vi "Locate Corner.vi"(7 "picture":refnum<vi>, 8 "error in":errorcluster, 9 "Corner Type":T1, 10 "Height":dbl=10000.0, 11 "color":string="Mat") -> (0 "error out":errorcluster, 2 "Robot Pose":cluster{"X":dbl, "Y":dbl, "Z":dbl, "A":dbl}, 3 "Robot Point":dbl[](array[numeric]), 5 "picture":picture)   [LabVIEW 2013]
uses:
  Teach Locations.ctl
  ROS/Code/SubVIs/BaxterSide.ctl
  <vilib>/Analysis/Matrix/Datatypes/RealMatrix.ctl
  <vilib>/Analysis/baseanly.llb/Mean (DBL).vi
  Arm Globals.vi
  Prim/Fwd Kenimatics - array.vi
  <vilib>/Analysis/Matrix/Numeric/Multiply/Multiply - RM,RM.vi
  ROS/Code/Console/Servers/ServerSubs/(nist) Arm Globals.vi
  Move/Move Axis.vi
  <vilib>/Analysis/Matrix/NI_Matrix.lvlib
  <vilib>/Analysis/NI_AALBase.lvlib
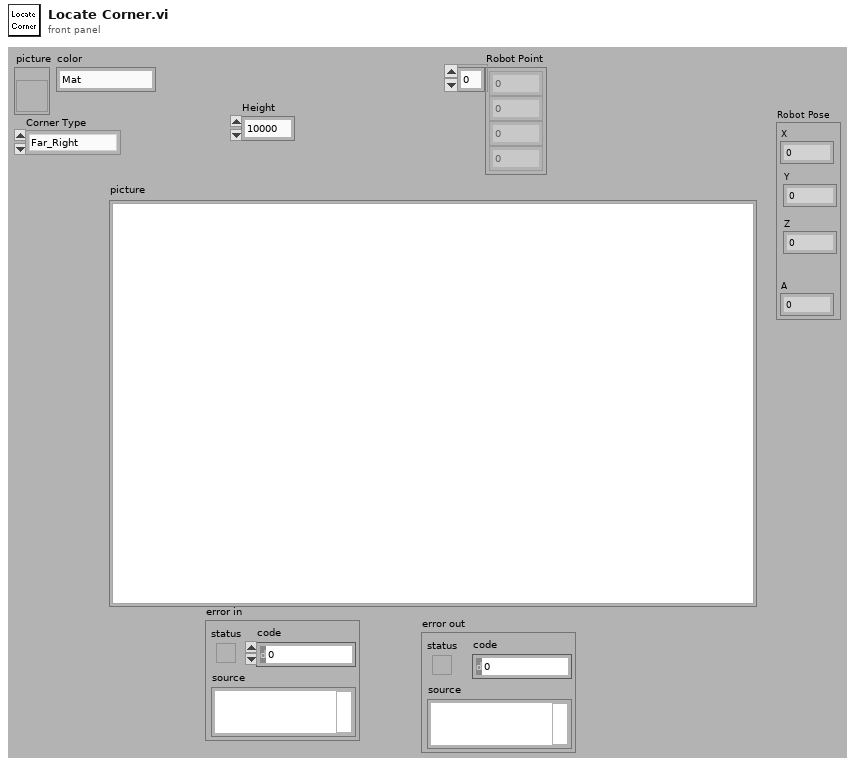
[diagram p1: front panel]
types:
  T1 = typedef "Teach Locations.ctl" = enum16{"Far_Right", "Near_Right", "Far_Left", "Near_Left", "Bottom", "Top", "Right", "Left"}
  T2 = cluster{"X":dbl, "Y":dbl, "Z":dbl, "O":dbl, "A":dbl, "T":dbl}
  T3 = typedef "BaxterSide.ctl" = enum16{"left", "right"}
  T4 = typedef "NI_Matrix.lvlib/RealMatrix.ctl" = dbl[][]
  T5 = cluster{"Real Matrix Element":dbl, "Real Matrix Element":dbl, "Real Matrix Element":dbl, "Real Matrix Element":dbl}
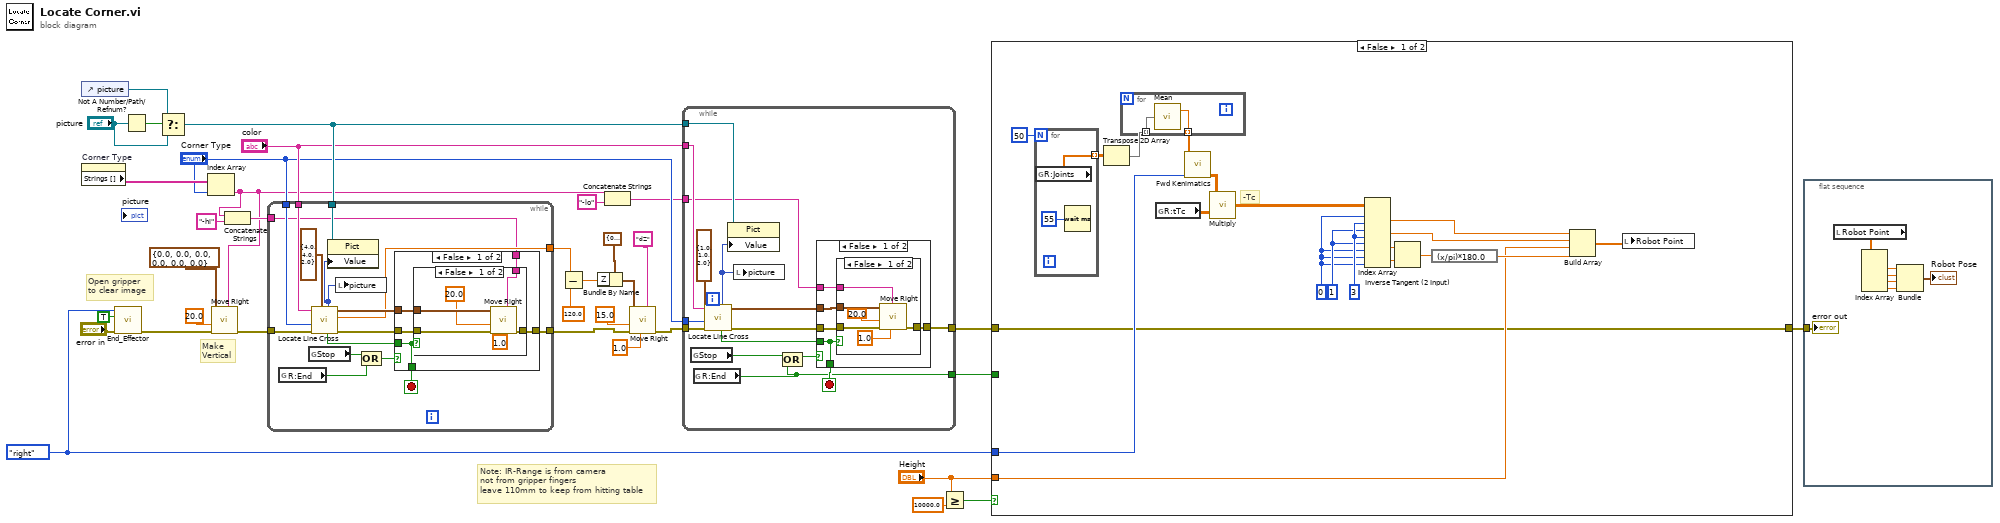
[diagram p0: block diagram]
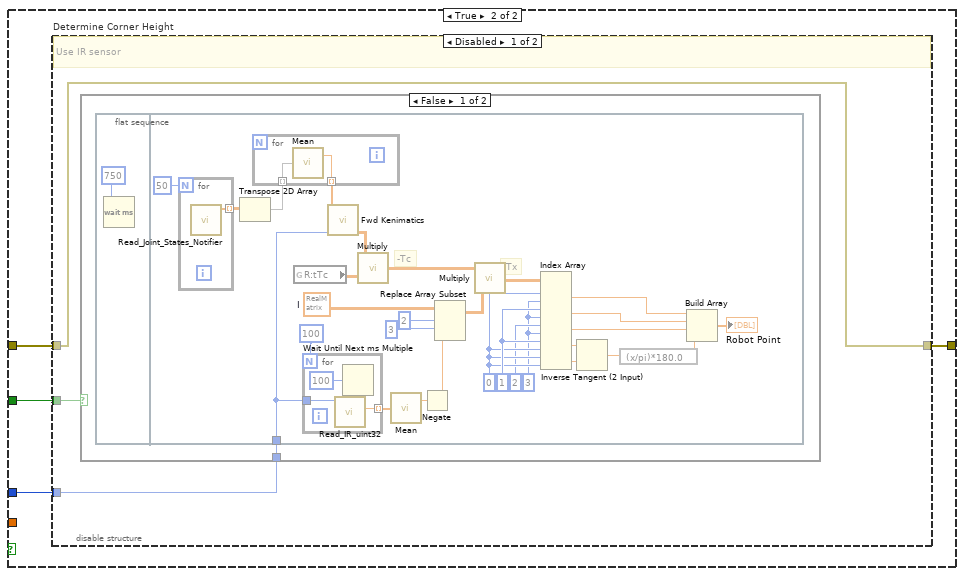
[diagram p2: hidden frame]
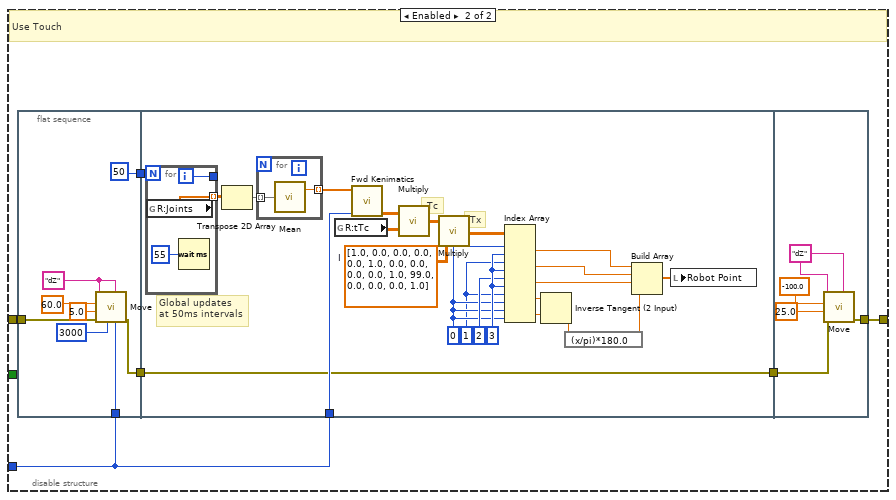
[diagram p4: hidden frame]
diagram:
  w23 = BaxterSide."right" ("Side")
  # "Make\nVertical"
  # "Open gripper\nto clear image"
  # "Note: IR-Range is from camera \nnot from gripper fingers\nleave 110mm to keep from hitting table"
  n1 = control-ref of="picture"() -> (w32:refnum<vi>)
  n2 = property on="Corner Type" class="Enum (strict)"() -> ("Strings []"=w25:string[])  [unwired: 2 in, 2 out]
  n3 = call "End_Effector.vi"("error in"="error in", "Close"=TRUE, "Side"=w23) -> ("error out"=w13:errorcluster)  [unwired: 5 in]
  n4 = Not A Number/Path/Refnum?(number/path/refnum="picture") -> (NaN/Path/Refnum?=w34:bool)
  n5 = Select(t=w32, s=w34, f="picture") -> (s? t:f=w35:refnum<vi>)
  n6 = Index Array(array=w25, index="Corner Type") -> (element=w10:string)
  n7 = call "Move Right.vi"("Label"=w10, "error in"=w13, "Speed (mm/s)"=20.0 ("Speed"), "Goal Axes"=T2 {"X"=0.0, "Y"=0.0, "Z"=0.0, "O"=0.0, "A"=0.0, "T"=0.0}) -> ("error out"=w12:errorcluster)  [unwired: 7 in]
  n8 = Concatenate Strings(w10, "-hi" ("string")) -> (w21:string)
  n9 = while {
    tunnel: w12 -> [w51]
    tunnel: [w49] -> w7
    tunnel: "color" -> [w39]
    tunnel: w35 -> [w43]
    tunnel: [w41] -> w27
    tunnel: "Corner Type" -> [w40]
    tunnel: w21 -> [w37]
    stop <- w45 stop-if-true
    n10 = global read "Arm Globals.vi" "R:End"() -> (w36:bool)
    n11 = global read "Arm Globals.vi" "Stop"() -> (w47:bool)
    n12 = call "Locate Line Cross.vi"("Tolerance"=cluster{"x":dbl, "y":dbl, "a":dbl} {"x"=4.0, "y"=4.0, "a"=2.0}, "error in"=w51, "Type"=w40, "color"=w39) -> ("error out"=w50:errorcluster, "Range"=w41:dbl, "result"=w48:T2, "Close"=w44:bool, "picture"=w38:picture)  [unwired: 2 in, 1 out]
    n13 = property class="Pict"(reference=w43, "Value"=w38) -> ()  [unwired: 1 in, 2 out]
    n14 = local write "picture"(w38) -> ()
    n15 = Compound Arithmetic op=OR(w47, w36) -> (w46:bool)
    n16 = case shown="False" w46 {
      selector: w46 -> [_ w64]
      tunnel: w50 -> [w56 w65]
      tunnel: [w55 w65] -> w49
      tunnel: w48 -> [w54 _]
      tunnel: [w53 w64] -> w45
      tunnel: w44 -> [w53 _]
      tunnel: w37 -> [w52 _]
      frame False {
        n17 = case shown="False" w53 {
          tunnel: w56 -> [w61 w63]
          tunnel: [w62 w63] -> w55
          tunnel: w54 -> [w58 _]
          tunnel: w52 -> [w60 _]
          frame False {
            n18 = call "Move Right.vi"("Label"=w60, "Wait Time"=1.0 ("wait time"), "error in"=w61, "Speed (mm/s)"=20.0 ("Speed"), "Goal Axes"=w58) -> ("error out"=w62:errorcluster)  [unwired: 6 in]
          }
          frame True {
          }
        }
      }
      frame True {
      }
    }
  }
  n19 = Subtract(x=w27, y=120.0) -> (x-y=w3:dbl)
  n20 = Bundle By Name(cluster=T2 {"X"=0.0, "Y"=0.0, "Z"=0.0, "O"=0.0, "A"=0.0, "T"=0.0} ("Goal Axes"), "Z"=w3) -> (w1:T2)
  n21 = Concatenate Strings(w10, "-lo" ("string")) -> (w19:string)
  n22 = call "Move Right.vi"("Label"="dZ" ("Location"), "Wait Time"=1.0 ("wait time"), "error in"=w7, "Speed (mm/s)"=15.0 ("Speed"), "Goal Axes"=w1) -> ("error out"=w8:errorcluster)  [unwired: 6 in]
  n23 = while {
    tunnel: w8 -> [w80]
    tunnel: [w78] -> w17
    tunnel: "color" -> [w75]
    tunnel: w35 -> [w71]
    tunnel: [w66] -> w29
    tunnel: "Corner Type" -> [w69]
    tunnel: w19 -> [w67]
    stop <- w72 stop-if-true
    n24 = global read "Arm Globals.vi" "Stop"() -> (w76:bool)
    n25 = global read "Arm Globals.vi" "R:End"() -> (w66:bool)
    n26 = call "Locate Line Cross.vi"("Tolerance"=cluster{"x":dbl, "y":dbl, "a":dbl} {"x"=1.0, "y"=1.0, "a"=2.0}, "error in"=w80, "Type"=w69, "color"=w75) -> ("error out"=w79:errorcluster, "result"=w77:T2, "Close"=w73:bool, "picture"=w68:picture)  [unwired: 2 in, 2 out]
    n27 = property class="Pict"(reference=w71, "Value"=w68) -> ()  [unwired: 1 in, 2 out]
    n28 = local write "picture"(w68) -> ()
    n29 = Compound Arithmetic op=OR(w76, w66) -> (w74:bool)
    n30 = case shown="False" w74 {
      selector: w74 -> [_ w93]
      tunnel: w73 -> [w82 _]
      tunnel: w79 -> [w85 w94]
      tunnel: [w84 w94] -> w78
      tunnel: w77 -> [w83 _]
      tunnel: [w82 w93] -> w72
      tunnel: w67 -> [w81 _]
      frame False {
        n31 = case shown="False" w82 {
          tunnel: w85 -> [w91 w92]
          tunnel: [w90 w92] -> w84
          tunnel: w83 -> [w88 _]
          tunnel: w81 -> [w87 _]
          frame False {
            n32 = call "Move Right.vi"("Label"=w87, "Wait Time"=1.0, "error in"=w91, "Speed (mm/s)"=20.0 ("Speed"), "Goal Axes"=w88) -> ("error out"=w90:errorcluster)  [unwired: 6 in]
          }
          frame True {
          }
        }
      }
      frame True {
      }
    }
  }
  n33 = Greater Or Equal?(x="Height", y=10000.0) -> (x >= y?=w15:bool)
  n34 = case shown="False" w15 {
    tunnel: w29 -> [_ w122]
    tunnel: w23 -> [w103 w121]
    tunnel: [w96 w120] -> w18
    tunnel: w17 -> [w96 w119]
    tunnel: "Height" -> [w101 _]
    frame False {
      w100 = 1 ("index (row)")
      w110 = 3 ("index (col)")
      w99 = 0 ("index (row)")
      # "-Tc"
      n35 = for {
        N: 50 -> [_]
        tunnel: [w118] -> w106 mode=indexing
        n36 = global read "(nist) Arm Globals.vi" "R:Joints"() -> (w118:dbl[])
        n37 = Wait (ms)(milliseconds to wait=u32 55) -> ()  [unwired: 1 out]
      }
      n38 = Transpose 2D Array(2D array=w106) -> (transposed array=w105:dbl[][])
      n39 = for {
        tunnel: w105 -> [w116] mode=indexing
        tunnel: [w115] -> w104 mode=indexing
        n40 = call-poly <vilib>:"Mean.vi"("X"=w116) -> ("mean"=w115:dbl)  [unwired: 1 out]
      }
      n41 = global read "Arm Globals.vi" "R:tTc"() -> (w108:T4)
      n42 = call-poly "Fwd Kenimatics.vi"("Side"=w103, "Joints"=w104) -> ("Matrix"=w109:T4)  [unwired: 8 in, 1 out]
      n43 = call-poly <vilib>:"Multiply.vi"("Real Matrix B"=w108, "Real Matrix A"=w109) -> ("A * B"=w102:T4)
      n44 = Index Array(array=w102, index (row) #1=w99, index (col) #1=w110, index (row) #2=w100, index (col) #2=w110, index (row) #3=w100, index (col) #3=w99, index (row) #4=w99, index (col) #4=w99) -> (element #1=w114:dbl, element #2=w113:dbl, element #3=w98:dbl, element #4=w97:dbl)
      n45 = Inverse Tangent (2 Input)(1:w97, 2:w98) -> (0:w111:dbl)
      n46 = expression code="(x/pi)*180.0" ("radians to degrees")(w111) -> (w112:dbl)
      n47 = Build Array(w114, w113, w101, w112) -> (w95:dbl[])
      n48 = local write "Robot Point"(w95) -> ()
    }
    frame True {
      n49 = disable-structure "Determine Corner Height" shown="Disabled" {
        disable-tunnel: w122 -> [w125 _]
        disable-tunnel: w121 -> [w124 w167]
        disable-tunnel: [w123 w165] -> w120
        disable-tunnel: w119 -> [w123 w168]
        frame Disabled {
          # "Use IR sensor"
          n50 = case shown="False" w125 {
            tunnel: w124 -> [w126 _]
            frame False {
              n51 = flat-sequence {
                tunnel: w126 -> [w132]
                frame #0 {
                  n52 = Wait (ms)(milliseconds to wait=u32 750) -> ()  [unwired: 1 out]
                }
                frame #1 {
                  w150 = 1 ("index (row)")
                  w145 = 3 ("index (col)")
                  w149 = 0 ("index (row)")
                  w139 = T4 [[1.0, 0.0, 0.0, 0.0], [0.0, 1.0, 0.0, 0.0], [0.0, 0.0, 1.0, 0.0], [0.0, 0.0, 0.0, 1.0]]  # I
                  # "-Tx"
                  # "-Tc"
                  n53 = for {
                    N: 50 -> [_]
                    tunnel: [w159] -> w130 mode=indexing
                    n54 = call "Read_Joint_States_Notifier.vi"() -> ("Positions"=w159:dbl[])  [unwired: 7 in, 1 out]
                  }
                  n55 = Transpose 2D Array(2D array=w130) -> (transposed array=w129:dbl[][])
                  n56 = for {
                    tunnel: w129 -> [w158] mode=indexing
                    tunnel: [w157] -> w128 mode=indexing
                    n57 = call-poly <vilib>:"Mean.vi"("X"=w158) -> ("mean"=w157:dbl)  [unwired: 1 out]
                  }
                  n58 = global read "Arm Globals.vi" "R:tTc"() -> (w134:T4)
                  n59 = for {
                    N: 100 -> [_]
                    tunnel: w132 -> [w162]
                    tunnel: [w161] -> w137 mode=indexing
                    n60 = call "Read_IR_uint32.vi"("Side"=w162) -> ("Distance"=w161:dbl)  [unwired: 4 in, 3 out]
                    n61 = Wait Until Next ms Multiple(millisecond multiple=u32 100) -> ()  [unwired: 1 out]
                  }
                  n62 = call-poly "Fwd Kenimatics.vi"("Side"=w132, "Joints"=w128) -> ("Matrix"=w135:T4)  [unwired: 8 in, 1 out]
                  n63 = call-poly <vilib>:"Multiply.vi"("Real Matrix B"=w134, "Real Matrix A"=w135) -> ("A * B"=w142:T4)
                  n64 = call-poly <vilib>:"Mean.vi"("X"=w137) -> ("mean"=w136:dbl)  [unwired: 1 out]
                  n65 = Negate(x=w136) -> (-x=w141:dbl)
                  n66 = Replace Array Subset(array=w139, new element=w141, index (row)=2 ("disabled index (row)"), index (col)=3 ("disabled index (col)")) -> (w143:T4)
                  n67 = call-poly <vilib>:"Multiply.vi"("Real Matrix B"=w143, "Real Matrix A"=w142) -> ("A * B"=w144:T4)
                  n68 = Index Array(array=w144, index (row) #1=w149, index (col) #1=w145, index (row) #2=w150, index (col) #2=w145, index (row) #3=2 ("index (row)"), index (col) #3=w145, index (row) #4=w150, index (col) #4=w149, index (row) #5=w149, index (col) #5=w149) -> (element #1=w155:dbl, element #2=w154:dbl, element #3=w153:dbl, element #4=w147:dbl, element #5=w148:dbl)
                  n69 = Inverse Tangent (2 Input)(1:w148, 2:w147) -> (0:w151:dbl)
                  n70 = expression code="(x/pi)*180.0" ("radians to degrees")(w151) -> (w152:dbl)
                  n71 = Build Array(w155, w154, w153, w152) -> (→"Robot Point":dbl[])
                }
              }
            }
            frame True {
            }
          }
        }
        frame Enabled {
          # "Use Touch"
          n72 = flat-sequence {
            tunnel: w168 -> [w176]
            tunnel: w167 -> [w172]
            tunnel: [50] -> w166
            tunnel: [w169] -> w164
            tunnel: w167 -> [w180]
            tunnel: w166 -> [w178]
            tunnel: w164 -> [w177]
            tunnel: [w177] -> w163
            tunnel: [w206] -> w165
            tunnel: w163 -> [w205]
            frame #0 {
              w174 = "dZ" ("Location")
              n73 = call-poly "Move.vi"("Side"=w172, "Label"=w174, "Wait Time"=3000, "error in"=w176, "Speed"=5.0 ("Speed (mm/s)"), "Value"=60.0 ("Speed (mm/s)"), "Location"=w174) -> ("error out"=w169:errorcluster)  [unwired: 4 in]
            }
            frame #1 {
              w186 = 1 ("index (row)")
              w191 = 3 ("index (col)")
              w187 = 0 ("index (row)")
              w199 = T4 [[1.0, 0.0, 0.0, 0.0], [0.0, 1.0, 0.0, 0.0], [0.0, 0.0, 1.0, 99.0], [0.0, 0.0, 0.0, 1.0]]  # I
              # "Global updates \nat 50ms intervals"
              # "-Tx"
              # "-Tc"
              n74 = for {
                N: w178 -> [_]
                tunnel: [w203] -> w196 mode=indexing
                tunnel: [w204] -> _
                i -> [w204]
                n75 = global read "(nist) Arm Globals.vi" "R:Joints"() -> (w203:dbl[])
                n76 = Wait (ms)(milliseconds to wait=u32 55) -> ()  [unwired: 1 out]
              }
              n77 = Transpose 2D Array(2D array=w196) -> (transposed array=w197:dbl[][])
              n78 = for {
                tunnel: w197 -> [w201] mode=indexing
                tunnel: [w200] -> w198 mode=indexing
                n79 = call-poly <vilib>:"Mean.vi"("X"=w201) -> ("mean"=w200:dbl)  [unwired: 1 out]
              }
              n80 = global read "Arm Globals.vi" "R:tTc"() -> (w195:T4)
              n81 = call-poly "Fwd Kenimatics.vi"("Side"=w180, "Joints"=w198) -> ("Matrix"=w194:T4)  [unwired: 8 in, 1 out]
              n82 = call-poly <vilib>:"Multiply.vi"("Real Matrix B"=w195, "Real Matrix A"=w194) -> ("A * B"=w193:T4)
              n83 = call-poly <vilib>:"Multiply.vi"("Real Matrix B"=w199, "Real Matrix A"=w193) -> ("A * B"=w192:T4)
              n84 = Index Array(array=w192, index (row) #1=w187, index (col) #1=w191, index (row) #2=w186, index (col) #2=w191, index (row) #3=2 ("index (row)"), index (col) #3=w191, index (row) #4=w186, index (col) #4=w187, index (row) #5=w187, index (col) #5=w187) -> (element #1=w181:dbl, element #2=w182:dbl, element #3=w183:dbl, element #4=w189:dbl, element #5=w188:dbl)
              n85 = Inverse Tangent (2 Input)(1:w188, 2:w189) -> (0:w185:dbl)
              n86 = expression code="(x/pi)*180.0" ("radians to degrees")(w185) -> (w184:dbl)
              n87 = Build Array(w181, w182, w183, w184) -> (w179:dbl[])
              n88 = local write "Robot Point"(w179) -> ()
            }
            frame #2 {
              w209 = "dZ" ("Location")
              n89 = call-poly "Move.vi"("Label"=w209, "error in"=w205, "Speed"=25.0 ("Speed (mm/s)"), "Value"=-100.0 ("Speed (mm/s)"), "Location"=w209) -> ("error out"=w206:errorcluster)  [unwired: 6 in]
            }
          }
        }
      }
    }
  }
  n90 = flat-sequence {
    tunnel: w18 -> [w216]
    frame #0 {
      n91 = local read "Robot Point"() -> (w214:dbl[])
      n92 = Index Array(array=w214) -> (element #1=w213:dbl, element #2=w212:dbl, element #3=w210:dbl, element #4=w211:dbl)  [unwired: 4 in]
      n93 = Bundle("Real Matrix Element"=w213, "Real Matrix Element"=w212, "Real Matrix Element"=w210, "Real Matrix Element"=w211) -> (→"Robot Pose":T5)  [unwired: 1 in]
      "error out" <- w216
    }
  }
